vi "실습 5-4.vi"() -> ()   [LabVIEW 2014]
panel:
  in  "머신 이름(\"\":  로컬 참조 열기)":string
  out "에러 출력":errorcluster
  in  "vi 경로":path
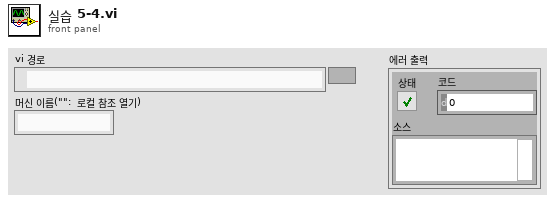
[diagram p1: front panel]
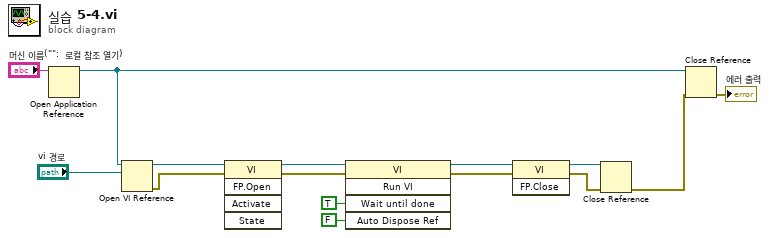
[diagram p0: block diagram]
diagram:
  n1 = Open Application Reference(11:"머신 이름(\"\":  로컬 참조 열기)") -> (3:w4:refnum<vi>)  [unwired: 3 in, 1 out]
  n2 = Open VI Reference(application reference (local)=w4, vi path="vi 경로") -> (vi reference=w14:refnum<vi>, error out=w10:errorcluster)  [unwired: 4 in]
  n3 = invoke class="VI" method="FP.Open"(reference=w14, error in=w10) -> (reference out=w13:refnum<vi>, error out=w11:errorcluster)  [unwired: 3 in, 3 out]
  n4 = invoke class="VI" method="Run VI"(reference=w13, error in=w11, "Wait until done"=TRUE ("완료될 때까지 기다림"), "Auto Dispose Ref"=FALSE ("참조 자동 삭제")) -> (reference out=w12:refnum<vi>, error out=w9:errorcluster)  [unwired: 1 in, 3 out]
  n5 = invoke class="VI" method="FP.Close"(reference=w12, error in=w9) -> (reference out=w6:refnum<vi>, error out=w5:errorcluster)  [unwired: 1 in, 1 out]
  n6 = Close Reference(reference=w6, error in (no error)=w5) -> (error out=w3:errorcluster)
  n7 = Close Reference(reference=w4, error in (no error)=w3) -> (error out=→"에러 출력":errorcluster)
